vi "Read DevId.vi"(8 "error in (no error)":errorcluster, 11 "Turn mTEC on in":refnum<class "Turn mTEC on.lvclass">) -> (0 "error out":errorcluster, 2 "DevId":string, 3 "Turn mTEC on out":refnum<class "Turn mTEC on.lvclass">)   [LabVIEW 2014, in "Controller.lvlib" / "Turn mTEC on.lvclass"]
uses:
  Turn mTEC on.lvclass
  Turn mTEC on.lvclass/Turn mTEC on.ctl
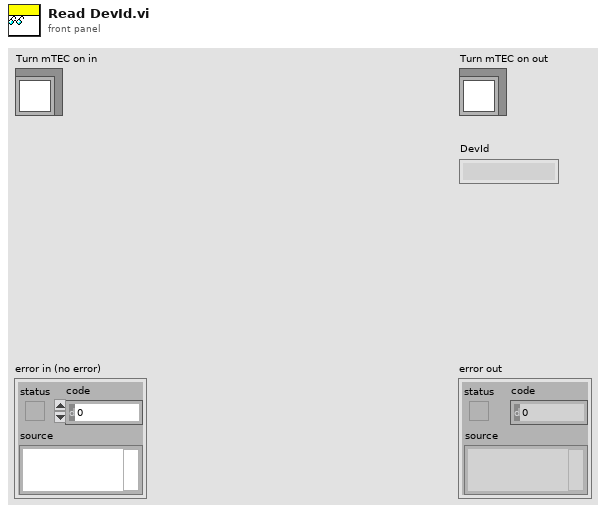
[diagram p1: front panel]
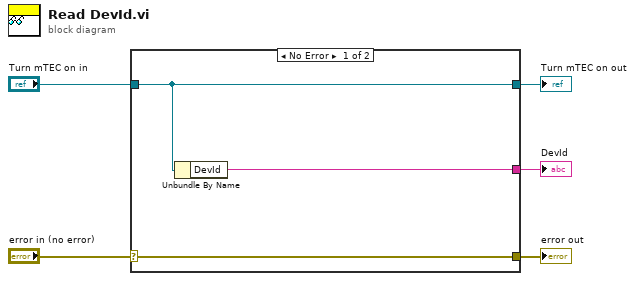
[diagram p0: block diagram]
diagram:
  n1 = case shown="No Error" "error in (no error)" {
    selector: "error in (no error)" -> [w8 w9]
    tunnel: [w8 w9] -> w4
    tunnel: [w7 w10] -> w2
    tunnel: "Turn mTEC on in" -> [w7 w10]
    tunnel: [w6 _] -> w1
    frame No Error {
      n2 = Unbundle By Name(w7) -> ("DevId"=w6:string)
    }
    frame Error {
    }
  }
  "error out" <- w4
  "Turn mTEC on out" <- w2
  "DevId" <- w1
